vi "DSF.Execution.Runtime.Plugin Manager.Find Plugin Classes.Runtime.vi"(8 "error in (no error)":errorcluster, 10 "Plugin objects":refnum<class>[](array[class]), 11 "Plugin Manager in":refnum<class "DSF.Engine.Runtime.Plugin Manager.lvclass">) -> (0 "error out":errorcluster, 2 "Plugin Runtime Classes":T1, 3 "Plugin Manager out":refnum<class "DSF.Engine.Runtime.Plugin Manager.lvclass">)   [LabVIEW 2017, in "DSF.Engine.lvlib" / "DSF.Engine.Runtime.Plugin Manager.lvclass"]
uses:
  DSF.Engine.Runtime.Plugin Manager.lvclass
  Shared/Typedefs/DSF.Shared.Typedefs.Plugin Classes.Runtime.ctl
  DSF.Shared.lvlib
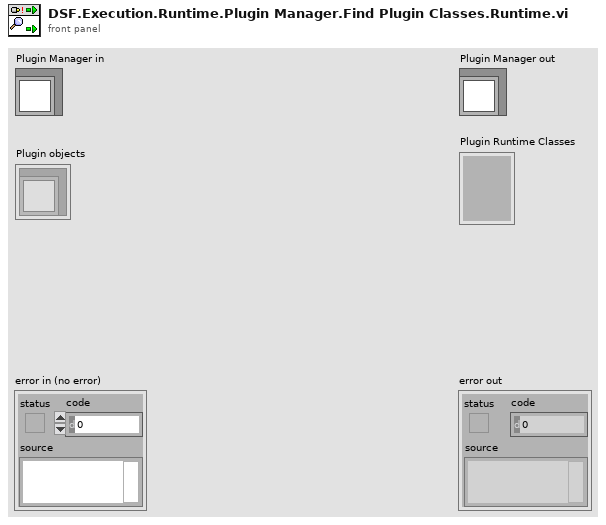
[diagram p1: front panel]
types:
  T1 = typedef "DSF.Shared.lvlib/DSF.Shared.Typedefs.Plugin Classes.Runtime.ctl" = cluster{}
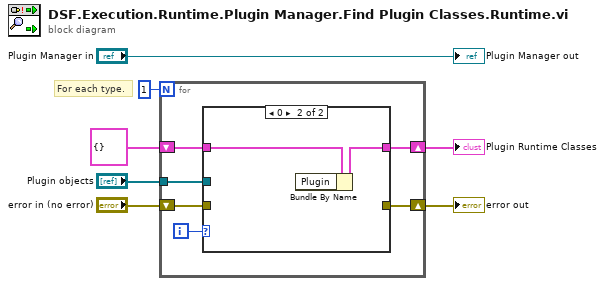
[diagram p0: block diagram]
diagram:
  # "For each type."
  n1 = for {
    N: 1 -> [_]
    shift-right: [w11] -> w2
    shift-left: T1 {} ("Plugin Runtime Classes") -> [w12]
    shift-right: [w10] -> w3
    shift-left: "error in (no error)" -> [w9]
    tunnel: "Plugin objects" -> [w8]
    i -> [w13]
    n2 = case shown="0" w13 {
      tunnel: w12 -> [w15 w17]
      tunnel: [w15 w16] -> w11
      tunnel: [w14 _] -> w10
      tunnel: w9 -> [w14 _]
      tunnel: w8 -> [_ _]
      frame -1, Default {
      }
      frame 0 {
        n3 = Bundle By Name(cluster=w17) -> (w16:T1)  [unwired: 1 in]
      }
    }
  }
  "error out" <- w3
  "Plugin Runtime Classes" <- w2
  "Plugin Manager out" <- "Plugin Manager in"
